vi "Conductance.vi"() -> ()   [LabVIEW 2021]
panel:
  out "Array - String":string[](array[string])
  out "Temperature vs scan number":cluster{dbl[], dbl[]}(graph)
  in  "Bacground resistance fraction":dbl
  in  "Temperature":string="Cryo-Con 32 (12) A"
  in  "Y":string="dIdV"
  in  "X":string="V"
  out "Scans":cluster{dbl[], dbl[]}[](graph)
  out "Scan temperatures":dbl[](array[numeric])
  in  "Scan indexes":i32[](array[numeric])=[1]
  in  "File Path":path=path "C:/Data/m010_072922.tdms"
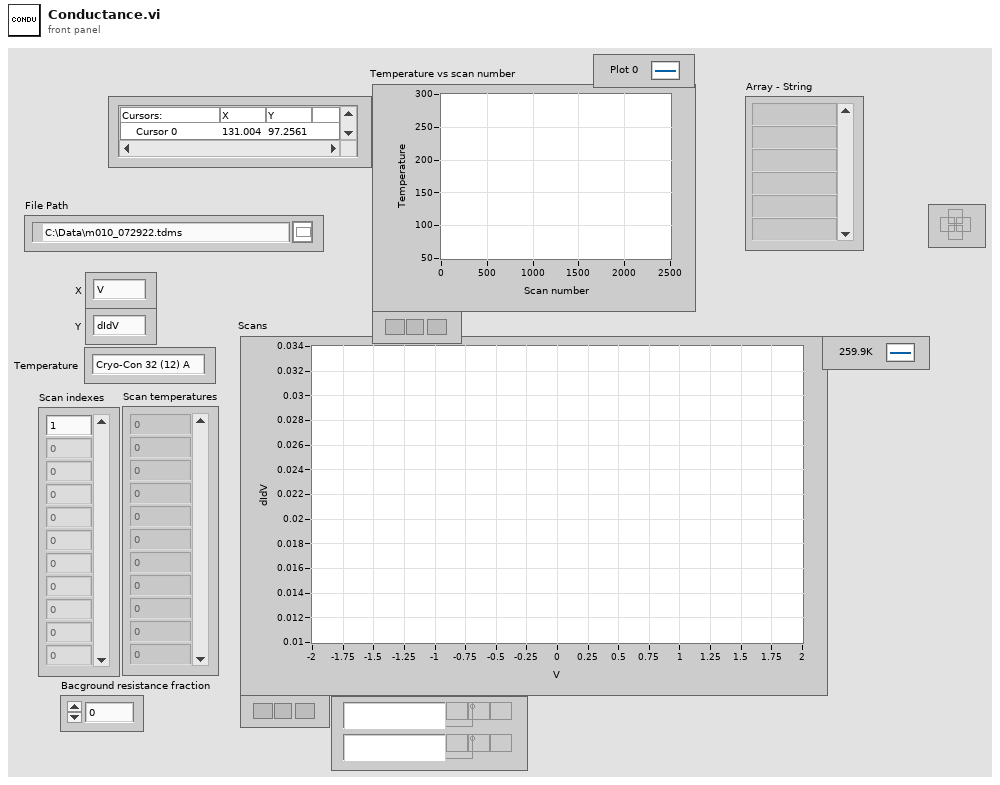
[diagram p1: front panel]
types:
  T1 = enum16{"open", "open or create", "create or replace", "create", "open (read-only)"}
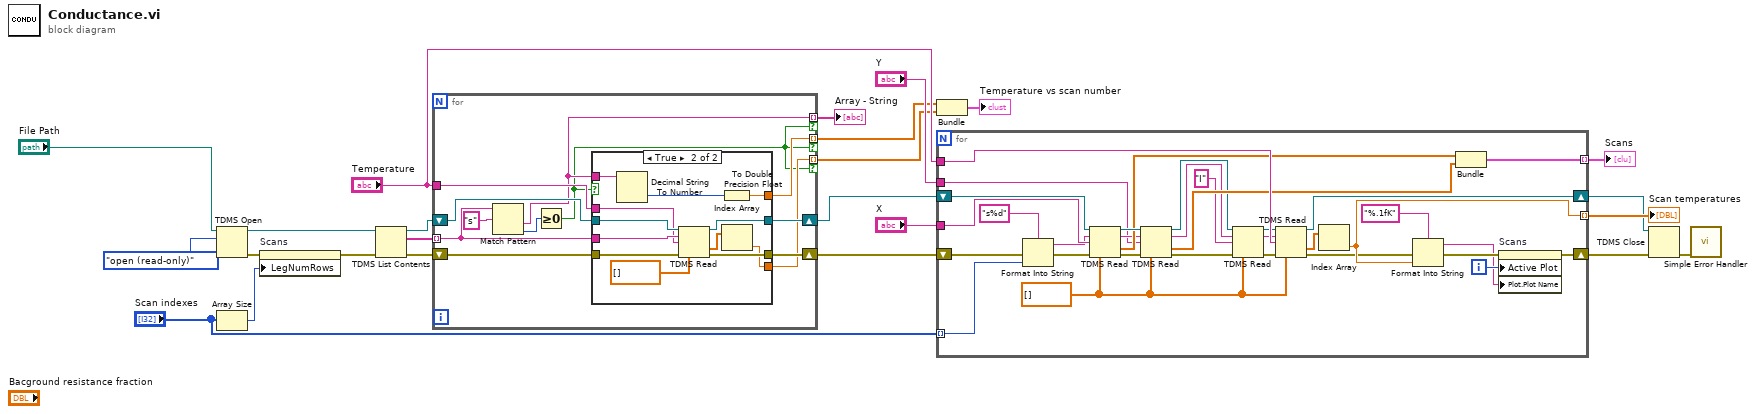
[diagram p0: block diagram]
diagram:
  n1 = TDMS Open(10:T1."open (read-only)" ("operation (0:open)"), 11:"File Path") -> (0:w15:errorcluster, 3:w9:refnum<k34>)  [unwired: 5 in]
  n2 = Array Size(array="Scan indexes") -> (size(s)=w16:i32)
  n3 = property on="Scans" class="XYGraph (strict)"(error in=w15, "LegNumRows"=w16) -> (error out=w8:errorcluster)  [unwired: 1 in, 1 out]
  n4 = TDMS List Contents(4:w8, 7:w9) -> (0:w11:errorcluster, 2:w12:string[], 3:w10:refnum<k34>)  [unwired: 1 in, 1 out]
  n5 = for {
    tunnel: w12 -> [w32] mode=indexing
    tunnel: [w27] -> w5 mode=indexing if=w25
    shift-right: [w30] -> w6
    shift-left: w10 -> [w34]
    shift-right: [w29] -> w7
    shift-left: w11 -> [w33]
    tunnel: "Temperature" -> [w31]
    tunnel: [w28] -> w1 mode=indexing if=w25
    tunnel: [w26] -> w2 mode=indexing if=w25
    n6 = Match Pattern(string=w32, regular expression="s") -> (after substring=w27:string, offset past match=w35:i32)  [unwired: 1 in, 2 out]
    n7 = Greater Or Equal To 0?(x=w35) -> (x >= 0?=w25:bool)
    n8 = case shown="True" w25 {
      tunnel: w34 -> [w38 w50]
      tunnel: w33 -> [w37 w49]
      tunnel: w32 -> [_ w47]
      tunnel: w31 -> [_ w46]
      tunnel: [w38 w45] -> w30
      tunnel: [w37 w44] -> w29
      tunnel: [_ w42] -> w28
      tunnel: w27 -> [_ w41]
      tunnel: [_ w39] -> w26
      frame False {
      }
      frame True {
        n9 = Decimal String To Number(string=w41) -> (number=w40:i32)  [unwired: 2 in, 1 out]
        n10 = TDMS Read(0:w50, 5:w47, 7:w46, 11:w49, 12:dbl[] []) -> (4:w45:refnum<k34>, 10:w43:dbl[], 15:w44:errorcluster)  [unwired: 3 in, 3 out]
        n11 = To Double Precision Float(number=w40) -> (double precision float=w39:dbl)
        n12 = Index Array(array=w43) -> (element=w42:dbl)  [unwired: 1 in]
      }
    }
  }
  "Array - String" <- w5
  n13 = Bundle(w2, w1) -> (→"Temperature vs scan number":cluster{dbl[], dbl[]})  [unwired: 1 in]
  n14 = for {
    tunnel: "Scan indexes" -> [w82] mode=indexing
    shift-right: [w69] -> w13
    shift-left: w7 -> [w80]
    tunnel: "Temperature" -> [w79]
    tunnel: [w66] -> w22 mode=indexing
    shift-right: [w52] -> w14
    shift-left: w6 -> [w63]
    tunnel: "X" -> [w72]
    tunnel: "Y" -> [w71]
    tunnel: [w70] -> w18 mode=indexing
    i -> [w67]
    w58 = dbl[] []
    n15 = Format Into String(format string="s%d", error in=w80, w82) -> (resulting string=w56:string, error out=w62:errorcluster)  [unwired: 1 in]
    n16 = TDMS Read(0:w63, 5:w56, 7:w72, 11:w62, 12:w58) -> (4:w76:refnum<k34>, 6:w73:string, 10:w75:dbl[], 15:w77:errorcluster)  [unwired: 3 in, 2 out]
    n17 = TDMS Read(0:w76, 5:w73, 7:w71, 11:w77, 12:w58) -> (4:w60:refnum<k34>, 6:w61:string, 10:w74:dbl[], 15:w59:errorcluster)  [unwired: 3 in, 2 out]
    n18 = TDMS Read(0:w60, 5:w61, 7:"I" ("channel name(s) in"), 11:w59, 12:w58) -> (4:w55:refnum<k34>, 6:w51:string, 15:w54:errorcluster)  [unwired: 3 in, 3 out]
    n19 = TDMS Read(0:w55, 5:w51, 7:w79, 11:w54, 12:w58) -> (4:w52:refnum<k34>, 10:w78:dbl[], 15:w53:errorcluster)  [unwired: 3 in, 3 out]
    n20 = Index Array(array=w78) -> (element=w66:dbl)  [unwired: 1 in]
    n21 = Format Into String(format string="%.1fK", error in=w53, w66) -> (resulting string=w64:string, error out=w68:errorcluster)  [unwired: 1 in]
    n22 = Bundle(w75, w74) -> (w70:cluster{dbl[], dbl[]})  [unwired: 1 in]
    n23 = property on="Scans" class="XYGraph (strict)"(error in=w68, "Active Plot"=w67, "Plot.Plot Name"=w64) -> (error out=w69:errorcluster)  [unwired: 1 in, 1 out]
  }
  "Scan temperatures" <- w22
  "Scans" <- w18
  n24 = TDMS Close(8:w13, 11:w14) -> (0:w21:errorcluster)  [unwired: 1 out]
  n25 = call <vilib>:"Simple Error Handler.vi"("error in (no error)"=w21) -> ()  [unwired: 4 in, 5 out]
